vi "Throw Error If Process Already in App.vi"(8 "error in (no error)":errorcluster, 10 "Process In":refnum<class "Process.lvclass">, 11 "Application In":refnum<class "Application.lvclass">) -> (0 "error out":errorcluster, 2 "Process Out":refnum<class "Process.lvclass">, 3 "Application Out":refnum<class "Application.lvclass">)   [LabVIEW 2020, in "Application.lvclass"]
uses:
  Application.lvclass
  Process/Process.lvclass
  <vilib>/Utility/error.llb/Error Cluster From Error Code.vi
  <vilib>/ErrorRing/Error Ring.xnode
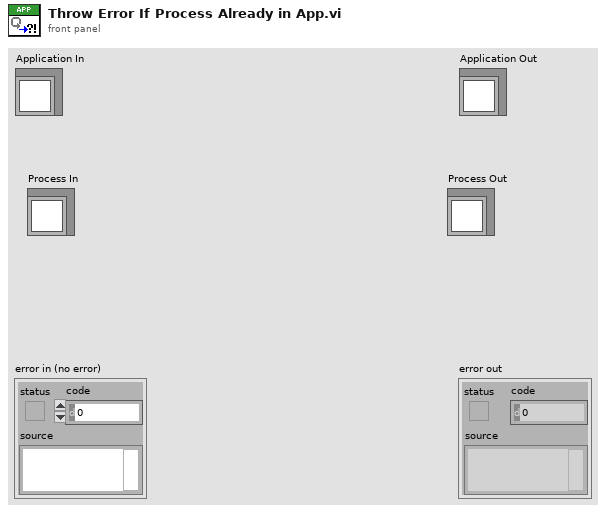
[diagram p1: front panel]
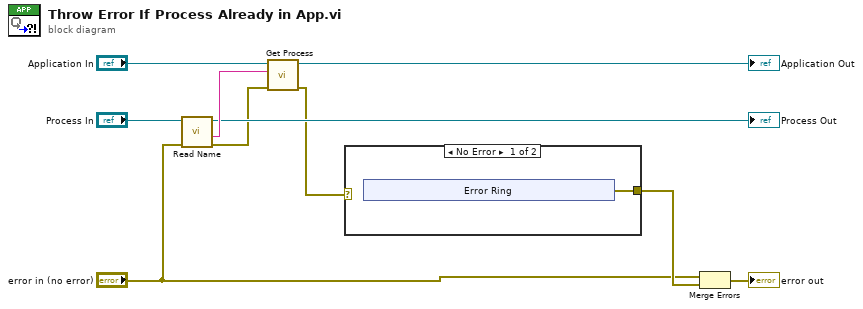
[diagram p0: block diagram]
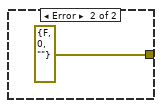
[diagram p2: hidden frame]
diagram:
  n1 = call-dynamic "Read Name.vi"("error in (no error)"="error in (no error)", "Process In"="Process In") -> ("error out"=w5:errorcluster, "Name"=w7:string, "Process Out"=→"Process Out":refnum<class "Process.lvclass">)  [unwired: 6 in, 1 out]
  n2 = call "Get Process.vi"("error in (no error)"=w5, "Process Name"=w7, "Rig In"="Application In") -> ("error out"=w4:errorcluster, "Rig Out"=→"Application Out":refnum<class "Application.lvclass">)  [unwired: 6 in, 1 out]
  n3 = case shown="No Error" w4 {
    tunnel: [w11 errorcluster {"status"=FALSE, "code"=0, "source"=""} ("error out")] -> w3
    frame No Error {
      n4 = xnode "Error Ring"() -> ("error out"=w11:errorcluster)
    }
    frame Error {
    }
  }
  n5 = Merge Errors("error in (no error)", w3) -> (→"error out":errorcluster)
